vi "Class_Custom Error.vi"(8 "error in":errorcluster) -> (0 "error out":errorcluster)   [LabVIEW 2020]
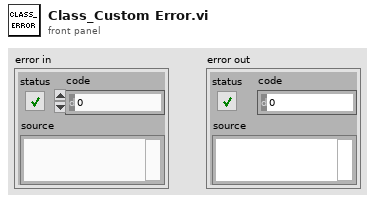
[diagram p1: front panel]
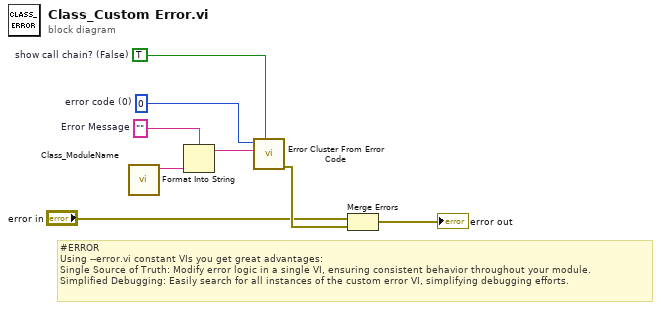
[diagram p0: block diagram]
diagram:
  w4 = 0  # error code (0)
  w2 = ""  # Error Message
  w5 = TRUE  # show call chain? (False)
  # "#ERROR\nUsing --error.vi constant VIs you get great advantages:\nSingle Source of Truth: Modify error logic in a single VI, ensuring consistent behavior throughout your module.\nSimplified Debugging: Easily search for all instances of the custom error VI, simplifying debugging efforts."
  n1 = call "Class_ModuleName.vi"() -> ("Module Name"=w1:string)  [unwired: 11 in]
  n2 = Format Into String(format string=w2, w1) -> (resulting string=w3:string)  [unwired: 2 in, 1 out]
  n3 = call <vilib>:"Error Cluster From Error Code.vi"("show call chain? (False)"=w5, "error message (\"\")"=w3, "error code (0)"=w4) -> ("error out"=w8:errorcluster)  [unwired: 6 in]
  n4 = Merge Errors("error in", w8) -> (→"error out":errorcluster)
